vi "15thermocluster.vi"() -> ()   [LabVIEW 2022 SP3]
panel:
  in  "Boolean":bool
  out "Array":T1(array[cluster])
  out "Temp Array":dbl[](array[numeric])
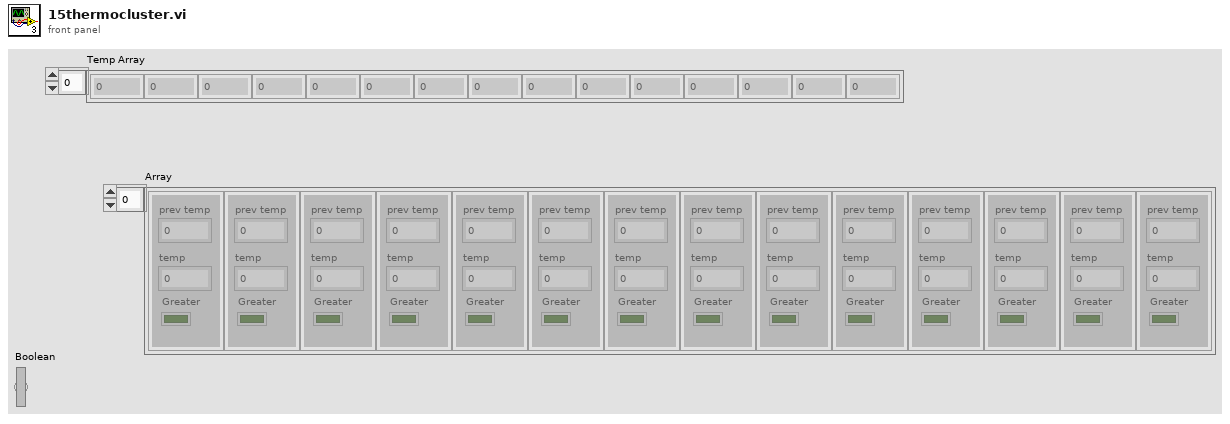
[diagram p1: front panel]
types:
  T1 = cluster{"prev temp":dbl, "temp ":dbl, "Greater":bool}[]
  T2 = cluster{"Thermometer":dbl, "Thermometer":dbl, bool}
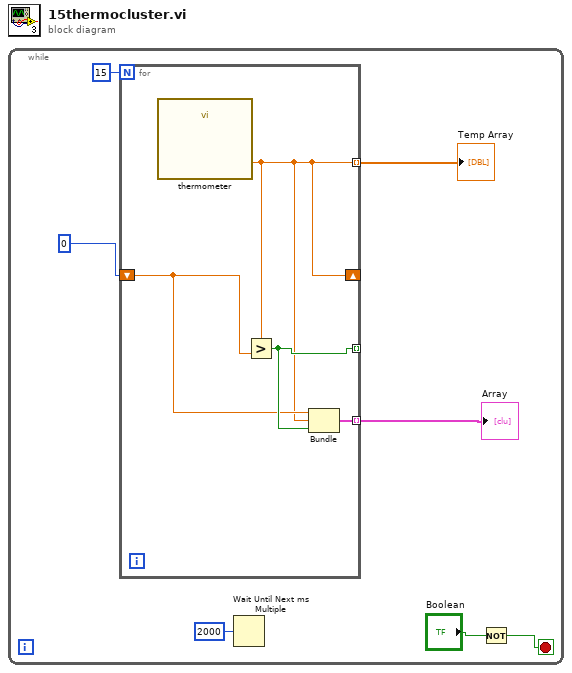
[diagram p0: block diagram]
diagram:
  n1 = while {
    stop <- w1 stop-if-true
    n2 = for {
      N: 15 -> [_]
      tunnel: [w9] -> w6 mode=indexing
      shift-right: [w9] -> _
      shift-left: 0 -> [w10]
      tunnel: [w11] -> _ mode=indexing
      tunnel: [w8] -> w5 mode=indexing
      n3 = call "thermometer.vi"() -> ("Thermometer"=w9:dbl)  [unwired: 1 in]
      n4 = Greater?(x=w9, y=w10) -> (0:w11:bool)
      n5 = Bundle("Thermometer"=w10, "Thermometer"=w9, w11) -> (w8:T2)  [unwired: 1 in]
    }
    "Temp Array" <- w6
    "Array" <- w5
    n6 = Wait Until Next ms Multiple(millisecond multiple=u32 2000) -> ()  [unwired: 1 out]
    n7 = Not(x="Boolean") -> (.not. x?=w1:bool)
  }
